vi "CoordAxis_U.vi"() -> (3 "out Coordinate Axis":T1)   [LabVIEW 2019, in "Trajectory_Library.lvlib"]
doc: "Convenience constructors that takes in x and y values directly instead of having to construct a Translation2d.\n\nParameters:\n - X- The x component of the translational component of the pose.\n - Y - The y component of the translational component of the pose.\n - Rotation (Heading) - The rotational component of the pose.\n\nReturns:\n - OUT POSE - Output POSE"
uses:
  COORDINATE_AXIS.ctl
  Trajectory_Library.lvlib
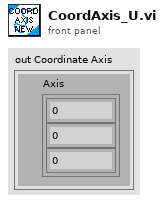
[diagram p1: front panel]
types:
  T1 = typedef "Trajectory_Library.lvlib/COORDINATE_AXIS.ctl" = cluster{"Axis":dbl[]}
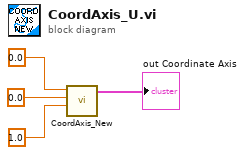
[diagram p0: block diagram]
diagram:
  n1 = call "CoordAxis_New.vi"("Z"=1.0, "Y"=0.0, "X"=0.0) -> ("out Coordinate Axis"=→"out Coordinate Axis":T1)  [unwired: 8 in]
